vi "Set Active User User Input.vi"(11 "Users":string[](array[string])) -> (0 "Date/Time":string, 3 "Selected User":string)   [LabVIEW 2016]
panel:
  in  "?":bool
  in  "Please find yourself in the list":string(combo)
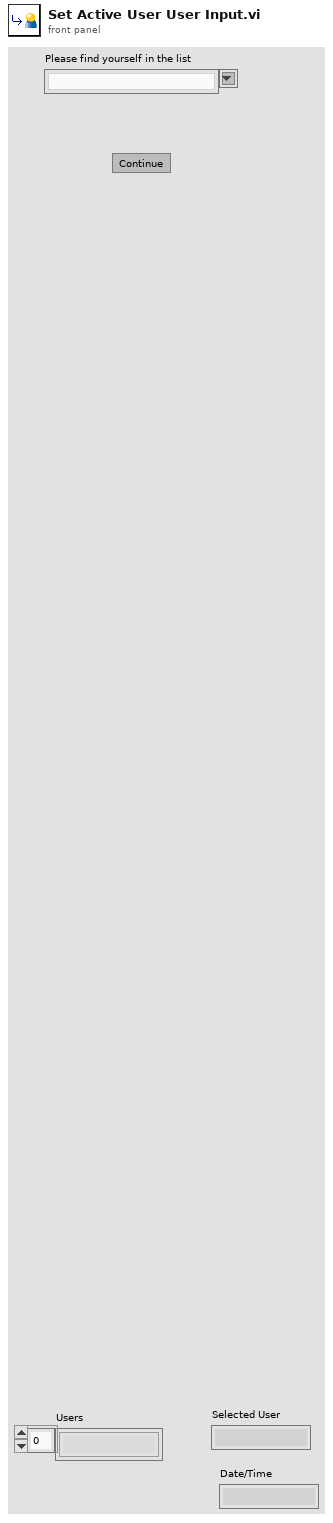
[diagram p1: front panel]
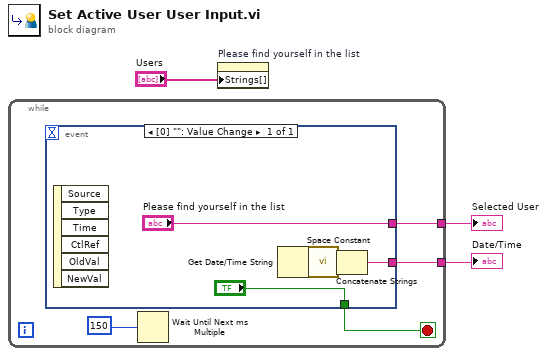
[diagram p0: block diagram]
diagram:
  n1 = while {
    tunnel: [w6] -> w2
    tunnel: [w4] -> w1
    stop <- w7 stop-if-true
    n2 = event shown="[0] \"\": Value Change" {
      selector: _ -> [_]
      dyn-events: _ -> [_]
      timeout: _ -> [_]
      tunnel: ["?"] -> w7
      tunnel: ["Please find yourself in the list"] -> w6
      tunnel: [w11] -> w4
      event Value Change {
        n3 = event-data() -> ()  [unwired: 1 in, 6 out]
        n4 = Get Date/Time String() -> (date string=w10:string, time string=w9:string)  [unwired: 3 in]
        n5 = call <vilib>:"Space Constant.vi"() -> ("String"=w8:string)
        n6 = Concatenate Strings(w10, w8, w9) -> (w11:string)
      }
    }
    n7 = Wait Until Next ms Multiple(millisecond multiple=150) -> ()  [unwired: 1 out]
  }
  "Selected User" <- w2
  "Date/Time" <- w1
  n8 = property on="Please find yourself in the list" class="CmbBox"("Strings[]"="Users") -> ()  [unwired: 2 in, 2 out]
